vi "Dispense FN - ON - Mass Loss (SubVI).vi"(0 "Measured Mass (g)":dbl, 3 "State Change?":bool, 5 "Measure Delay Complete?":bool) -> (17 "Dispense Mass Loss":dbl)   [LabVIEW 2009]
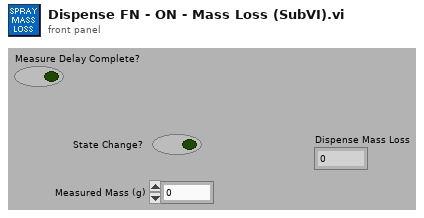
[diagram p1: front panel]
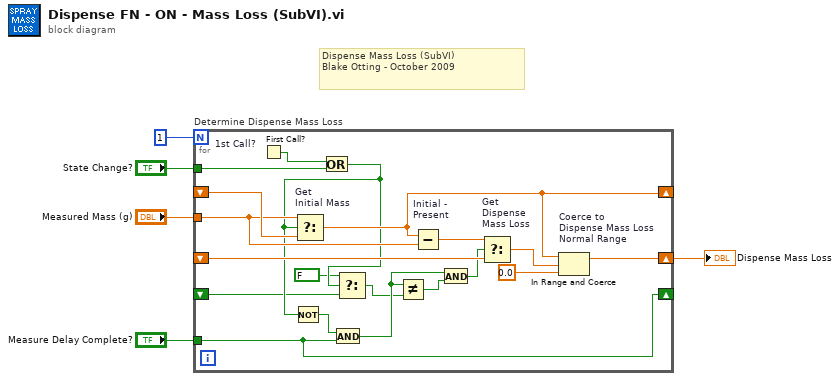
[diagram p0: block diagram]
diagram:
  # "Dispense Mass Loss (SubVI)\nBlake Otting - October 2009"
  n1 = for "Determine Dispense Mass Loss" {
    N: 1 -> [_]
    tunnel: "Measured Mass (g)" -> [w18]
    shift-right: [w19] -> _
    shift-left: _ -> [w24]
    shift-right: [w17] -> w5
    shift-left: _ -> [w23]
    tunnel: "State Change?" -> [w15]
    shift-right: [w6] -> _
    shift-left: _ -> [w9]
    tunnel: "Measure Delay Complete?" -> [w6]
    n2 = First Call? "1st Call?"() -> (First Call?: T/F=w7:bool)
    n3 = Or(x=w7, y=w15) -> (x .or. y?=w11:bool)
    n4 = Not(x=w11) -> (.not. x?=w13:bool)
    n5 = Select "Get\nInitial Mass"(t=w18, s=w11, f=w24) -> (s? t:f=w19:dbl)
    n6 = And(x=w13, y=w6) -> (x .and. y?=w12:bool)
    n7 = Select(t=FALSE, s=w11, f=w9) -> (s? t:f=w8:bool)
    n8 = Not Equal?(x=w12, y=w8) -> (x != y?=w16:bool)
    n9 = Subtract "Initial -\nPresent"(x=w19, y=w18) -> (x-y=w22:dbl)
    n10 = And(x=w12, y=w16) -> (x .and. y?=w14:bool)
    n11 = Select "Get\nDispense\nMass Loss"(t=w22, s=w14, f=w23) -> (s? t:f=w20:dbl)
    n12 = In Range and Coerce "Coerce to\nDispense Mass Loss \nNormal Range"(upper limit=w19, x=w20, lower limit=0.0) -> (coerced(x)=w17:dbl)  [unwired: 1 out]
  }
  "Dispense Mass Loss" <- w5
